vi "Close (Filter).vi"(8 "error in (no error)":errorcluster, 11 "Filter in":refnum<k20>) -> (0 "error out":errorcluster)   [LabVIEW 2020, in "nisyscfg.lvlib"]
doc: "Closes a reference to a system filter."
uses:
  <vilib>/nisyscfg/nisyscfg.lvlib
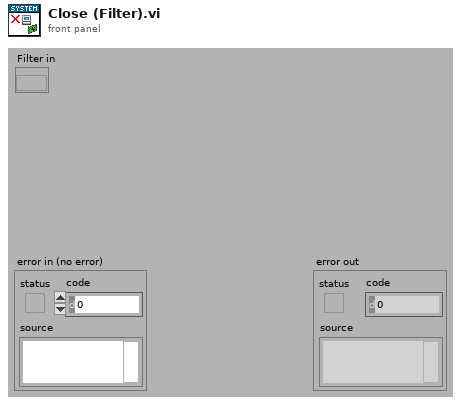
[diagram p1: front panel]
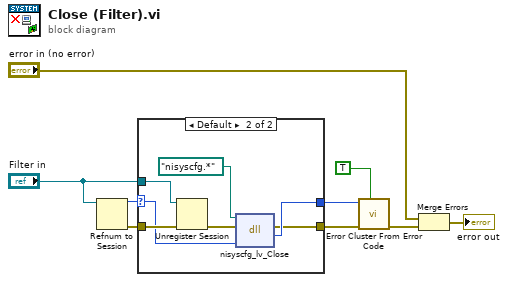
[diagram p0: block diagram]
diagram:
  n1 = Refnum to Session(7:"Filter in") -> (0:w2:errorcluster, 3:w1:u64)  [unwired: 1 in]
  n2 = case shown="Default" w1 {
    selector: w1 -> [_ w11]
    tunnel: "Filter in" -> [_ w17]
    tunnel: [_ w16] -> w5
    tunnel: [w10 w15] -> w4
    tunnel: w2 -> [w10 w12]
    frame 0 {
      # "Closing an invalid refnum\nor closing twice is wrong.\nBut returning an error would\nbreak compatibility."
    }
    frame Default {
      n3 = Unregister Session(8:w12, 11:w17) -> (0:w13:errorcluster)
      n4 = dll-call lib="nisyscfg.*" fn="nisyscfg_lv_Close" label="Close"(path in=path "nisyscfg.*", error in=w13, "filter"=w11) -> (error out=w15:errorcluster, "status"=w16:i32)  [unwired: 1 in, 2 out]
    }
  }
  n5 = call <vilib>:"Error Cluster From Error Code.vi"("show call chain? (False)"=TRUE, "error in (no error)"=w4, "error code (0)"=w5) -> ("error out"=w6:errorcluster)  [unwired: 6 out]
  n6 = Merge Errors("error in (no error)", w6) -> (→"error out":errorcluster)
